vi "NR Configure CHP.vi"(0 "RFmx Handle In":refnum<k21>, 1 "Selector String":string, 5 "NR CHP Configuration":T1={"Sweep Time Auto"=1, "Sweep Time Interval (s)"=0.001, "Averaging Enabled"=0, "Averaging Count"=10, "Averaging Type"=0} {"Sweep Time Auto" items=["False", "True"]; "Averaging Type" items=["RMS", "Log", "Scalar", "Max", "Min"]; "Averaging Enabled" items=["False", "True"]}, 11 "error in (no error)":errorcluster) -> (4 "RFmx Handle Out":refnum<k21>, 15 "error out":errorcluster)   [LabVIEW 2019, in "RFmxNR.lvlib"]
doc: "Configures common settings for the CHP measurement and selects the measurement."
uses:
  RFmxNR.lvlib
  Typedefs/NR CHP Configuration.ctl
  <vilib>/RFmx/NR/mx/RFmxNR.llb/RFmxNR Select Measurement (Single).vi
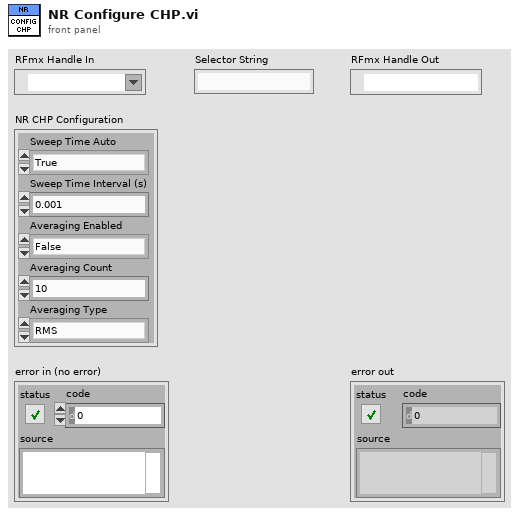
[diagram p1: front panel]
types:
  T1 = typedef "RFmxNR.lvlib/NR CHP Configuration.ctl" = cluster{"Sweep Time Auto":i32, "Sweep Time Interval (s)":dbl, "Averaging Enabled":i32, "Averaging Count":i32, "Averaging Type":i32}
  T2 = enum16{"ModAcc", "SEM", "ACP", "CHP", "OBW", "PVT"}
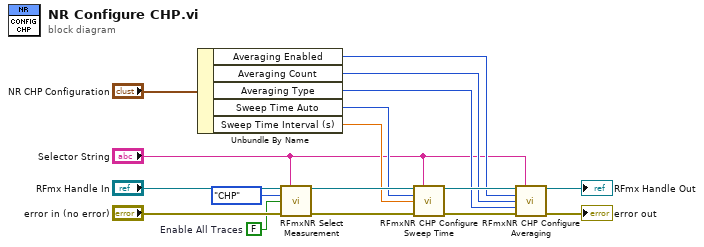
[diagram p0: block diagram]
diagram:
  w1 = FALSE  # Enable All Traces
  n1 = Unbundle By Name("NR CHP Configuration") -> ("Averaging Enabled"=w7:i32, "Averaging Count"=w6:i32, "Averaging Type"=w5:i32, "Sweep Time Auto"=w9:i32, "Sweep Time Interval (s)"=w8:dbl)
  n2 = call-poly <vilib>:"RFmxNR Select Measurement.vi"("Instrument Handle In"="RFmx Handle In", "Selector String"="Selector String", "Measurement"=T2."CHP", "Enable All Traces"=w1, "error in (no error)"="error in (no error)") -> ("Instrument Handle Out"=w16:refnum<k21>, "error out"=w12:errorcluster)  [unwired: 9 in]
  n3 = call <vilib>:"RFmxNR CHP Configure Sweep Time.vi"("Instrument Handle In"=w16, "Selector String"="Selector String", "Sweep Time Auto"=w9, "Sweep Time Interval (s)"=w8, "error in (no error)"=w12) -> ("Instrument Handle Out"=w15:refnum<k21>, "error out"=w11:errorcluster)  [unwired: 9 in]
  n4 = call <vilib>:"RFmxNR CHP Configure Averaging.vi"("Instrument Handle In"=w15, "Selector String"="Selector String", "Averaging Enabled"=w7, "Averaging Count"=w6, "Averaging Type"=w5, "error in (no error)"=w11) -> ("Instrument Handle Out"=→"RFmx Handle Out":refnum<k21>, "error out"=→"error out":errorcluster)  [unwired: 8 in]
